vi "Get Neighbor Values.vi"(10 "neighbor coordinates":i32[][](array[numeric]), 11 "cells in":bool[][](array[boolean])) -> (3 "cells living":bool[](array[boolean]))   [LabVIEW 2021, in "Game of Life.lvlib"]
doc: "This VI gets the boolean values of the neighbor cells."
uses:
  Game of Life.lvlib
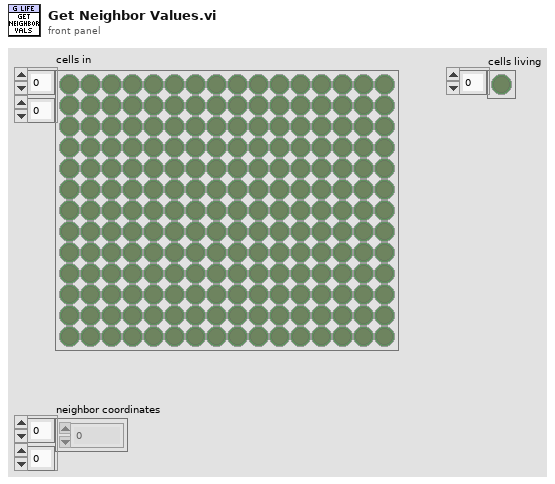
[diagram p1: front panel]
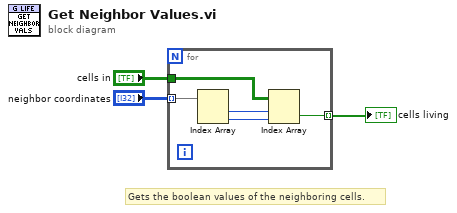
[diagram p0: block diagram]
diagram:
  # "Gets the boolean values of the neighboring cells."
  n1 = for {
    tunnel: "neighbor coordinates" -> [w8] mode=indexing
    tunnel: "cells in" -> [w5]
    tunnel: [w4] -> w1 mode=indexing
    n2 = Index Array(array=w8) -> (element #1=w7:i32, element #2=w6:i32)  [unwired: 2 in]
    n3 = Index Array(array=w5, index (row)=w7, index (col)=w6) -> (element=w4:bool)
  }
  "cells living" <- w1
